vi "DBConnect-Com-Exec.vi"(8 "error in (no error)":errorcluster, 9 "ControlQueue":refnum<queue>, 10 "data":variant, 11 "DB in":refnum<class "DB.lvclass">) -> (0 "error out":errorcluster, 3 "DB out":refnum<class "DB.lvclass">)   [LabVIEW 2019, in "DB.lvclass"]
uses:
  DB.lvclass
  C:/Users/elysium/Documents/dev/TRANCON/Classes/GeneralFunctionality/GeneralFunctionality.lvclass
  dependecies/ControlsVIs/Clusters-def/SERVER-Commands.ctl
  dependecies/ControlsVIs/Clusters-def/DB-Reply-to-Connect.ctl
  dependecies/ControlsVIs/Clusters-def/DB-Reply-Connect-Client.ctl
  GeneralFunctionality/GeneralFunctionality.lvclass/GeneralFunctionality.ctl
  Control/Control-Server/Control-Server.lvclass
  GeneralFunctionality/GeneralFunctionality.lvclass
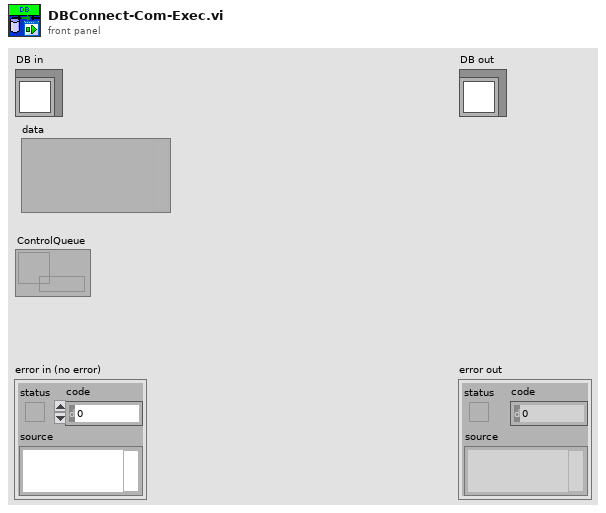
[diagram p1: front panel]
types:
  T1 = typedef "Control-Server.lvclass/SERVER-Commands.ctl" = string
  T2 = typedef "DB.lvclass/DB-Reply-Connect-Client.ctl" = cluster{"on/off":bool, "error":errorcluster}
  T3 = typedef "DB.lvclass/DB-Reply-to-Connect.ctl" = cluster{"On/Off":bool, "error":errorcluster, "DB.lvclass":refnum<class "DB.lvclass">}
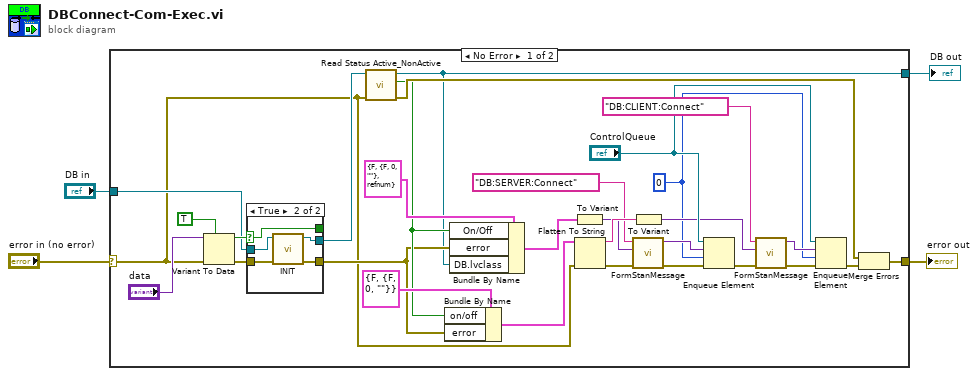
[diagram p0: block diagram]
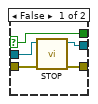
[diagram p2: hidden frame]
diagram:
  n1 = case shown="No Error" "error in (no error)" {
    selector: "error in (no error)" -> [w19 w46]
    tunnel: [w27 w46] -> w4
    tunnel: [w5 w45] -> w3
    tunnel: "DB in" -> [w30 w45]
    frame No Error {
      w6 = 0 ("timeout en ms (-1)")
      n2 = Variant To Data(error in=w19, type=TRUE, Variant="data") -> (data=w32:bool, error out=w31:errorcluster)
      n3 = case shown="True" w32 {
        selector: w32 -> [w35 w44]
        tunnel: w31 -> [w39 w40]
        tunnel: w30 -> [w37 w41]
        tunnel: [w36 w42] -> w25
        tunnel: [w38 w43] -> w22
        tunnel: [w35 w44] -> _
        frame False {
          n4 = call-dynamic "STOP.vi"("error in (no error)"=w39, "Stop in"=w37) -> ("error out"=w38:errorcluster, "Stop out"=w36:refnum<class "DB.lvclass">)  [unwired: 8 in]
        }
        frame True {
          n5 = call-dynamic "INIT.vi"("error in (no error)"=w40, "GeneralFunctionality in"=w41) -> ("error out"=w43:errorcluster, "GeneralFunctionality out"=w42:refnum<class "DB.lvclass">)  [unwired: 8 in]
        }
      }
      n6 = call "Read Status Active_NonActive.vi"("error in (no error)"=w19, "GeneralFunctionality in"=w25) -> ("error out"=w28:errorcluster, "Status Active/NonActive"=w23:bool, "GeneralFunctionality out"=w5:refnum<class "DB.lvclass">)  [unwired: 7 in]
      n7 = Bundle By Name(cluster=T2 {"on/off"=FALSE, "error"={"status"=FALSE, "code"=0, "source"=""}} ("output cluster"), "on/off"=w23, "error"=w22) -> (w21:T2)
      n8 = Bundle By Name(cluster=T3 {"On/Off"=FALSE, "error"={"status"=FALSE, "code"=0, "source"=""}, "DB.lvclass"=refnum} ("Cluster"), "On/Off"=w23, "error"=w22, "DB.lvclass"=w5) -> (w29:T3)
      n9 = To Variant(anything=w29) -> (Variant=w9:variant)
      n10 = Flatten To String(anything=w21, error in (no error)=w19) -> (data string=w20:string, error out=w17:errorcluster)  [unwired: 2 in, 1 out]
      n11 = call "FormStanMessage.vi"("error in"=w17, "data"=w9, "Command"=T1 "DB:SERVER:Connect" ("Commands")) -> ("error out"=w16:errorcluster, "message"=w15:variant)  [unwired: 7 in]
      n12 = To Variant(anything=w20) -> (Variant=w7:variant)
      n13 = Enqueue Element(queue="ControlQueue", element=w15, timeout in ms (-1)=w6, error in (no error)=w16) -> (error out=w14:errorcluster)  [unwired: 2 out]
      n14 = call "FormStanMessage.vi"("error in"=w14, "data"=w7, "Command"=T1 "DB:CLIENT:Connect" ("Commands")) -> ("error out"=w13:errorcluster, "message"=w8:variant)  [unwired: 7 in]
      n15 = Enqueue Element(queue="ControlQueue", element=w8, timeout in ms (-1)=w6, error in (no error)=w13) -> (error out=w12:errorcluster)  [unwired: 2 out]
      n16 = Merge Errors(w28, w12) -> (w27:errorcluster)
    }
    frame Error {
    }
  }
  "error out" <- w4
  "DB out" <- w3
